vi "Parse Payload File.vi"(8 "error in":errorcluster, 11 "frame array path in":path caption="path to parameters xml") -> (0 "error out":errorcluster, 2 "Map":T1 {"value"."Type of Frame" items=["Raw Frame", "UDP/IP Tx Gen", "Tx UDP"]; "value"."Data" format="%.0x"}, 3 "frame array path out":path caption="path to parameters xml")   [LabVIEW 2020, in "AIM ARINC 664 Scripting.lvlib"]
uses:
  AIM ARINC 664 Scripting.lvlib
  Frame Configuration/controls/Type of Payload.ctl
  Frame Configuration/controls/Payload Record Type.ctl
  Frame Configuration/controls/Payload Map.ctl
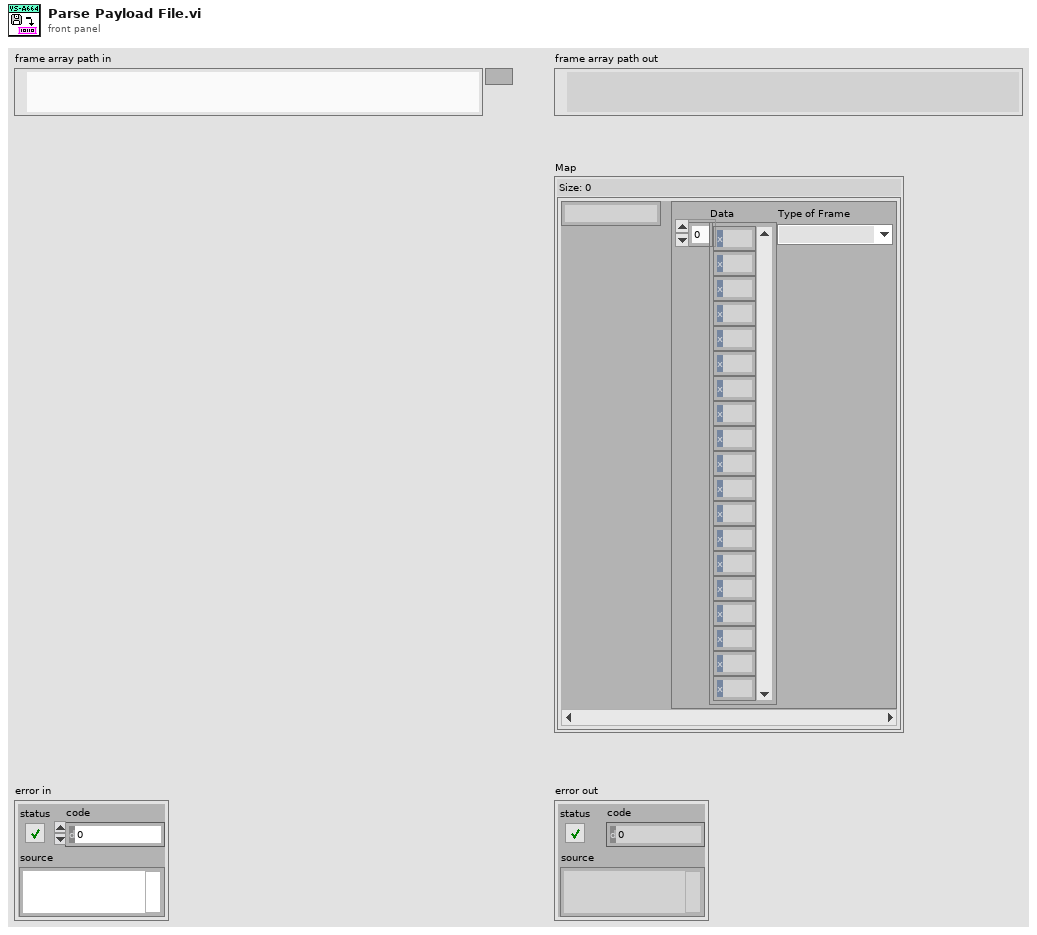
[diagram p1: front panel]
types:
  T1 = typedef "Payload Map.ctl" = map{string, T2}
  T2 = typedef "Payload Record Type.ctl" = cluster{"Data":u8[], "Type of Frame":T3}
  T3 = typedef "Type of Payload.ctl" = u16
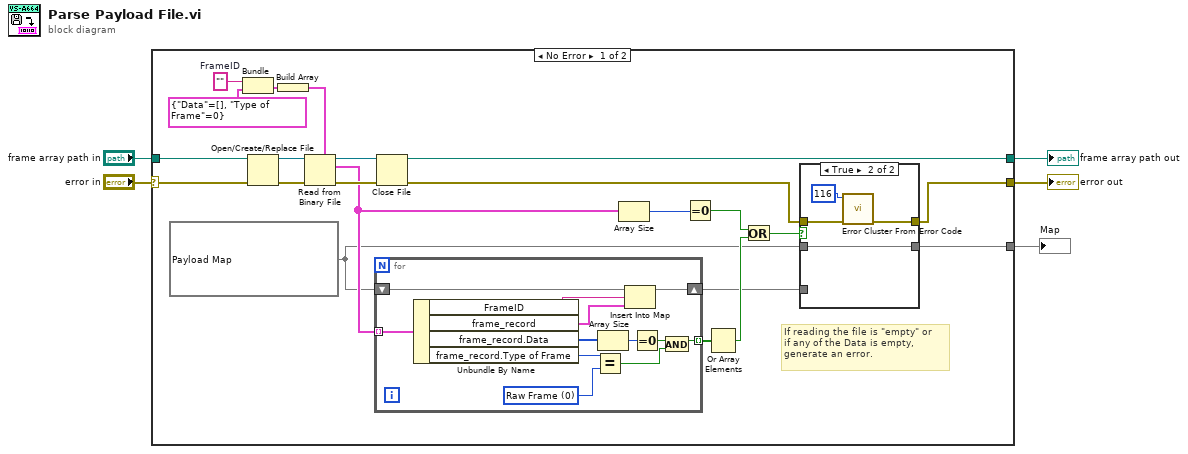
[diagram p0: block diagram]
diagram:
  n1 = case shown="No Error" "error in" {
    selector: "error in" -> [w22 w47]
    tunnel: [w15 w47] -> w5
    tunnel: "frame array path in" -> [w24 w46]
    tunnel: [w23 w46] -> w2
    tunnel: [w7 _] -> w1
    frame No Error {
      w20 = ""  # FrameID
      w6 = T1 {}
      # "If reading the file is \"empty\" or \nif any of the Data is empty,\ngenerate an error."
      n2 = Bundle("FrameID"=w20, "frame_record"=T2 {"Data"=[], "Type of Frame"=0}) -> (w21:cluster{"FrameID":string, "frame_record":T2})  [unwired: 1 in]
      n3 = Open/Create/Replace File(file path (use dialog)=w24, error in=w22) -> (refnum out=w26:refnum<file>, error out=w27:errorcluster)  [unwired: 4 in, 1 out]
      n4 = Build Array(w21) -> (w18:cluster{"FrameID":string, "frame_record":T2}[])
      n5 = Read from Binary File(5:w18, 8:w27, 11:w26) -> (0:w17:errorcluster, 2:w14:cluster{"FrameID":string, "frame_record":T2}[], 3:w25:refnum<file>)  [unwired: 3 in, 1 out]
      n6 = for {
        shift-right: [w44] -> w8
        shift-left: w6 -> [w45]
        tunnel: w14 -> [w41] mode=indexing
        tunnel: [w35] -> w10 mode=indexing
        w36 = T3 0 items=["Raw Frame", "UDP/IP Tx Gen", "Tx UDP"] ("y")
        n7 = Unbundle By Name(w41) -> ("FrameID"=w43:string, "frame_record"=w42:T2, "frame_record.Data"=w40:u8[], "frame_record.Type of Frame"=w37:T3)
        n8 = Equal?(x=w37, y=w36) -> (x = y?=w34:bool)
        n9 = Array Size(array=w40) -> (size(s)=w39:i32)
        n10 = Insert Into Map(map in=w45, key=w43, value=w42) -> (map out=w44:T1)  [unwired: 2 out]
        n11 = Equal To 0?(x=w39) -> (x = 0?=w38:bool)
        n12 = And(x=w38, y=w34) -> (x .and. y?=w35:bool)
      }
      n13 = Close File(refnum=w25, error in=w17) -> (path=w23:path, error out=w16:errorcluster)
      n14 = Array Size(array=w14) -> (size(s)=w13:i32)
      n15 = Equal To 0?(x=w13) -> (x = 0?=w12:bool)
      n16 = Or Array Elements(Boolean array=w10) -> (logical OR=w9:bool)
      n17 = Or(x=w12, y=w9) -> (x .or. y?=w11:bool)
      n18 = case shown="True" w11 {
        tunnel: w16 -> [w29 w33]
        tunnel: [w29 w32] -> w15
        tunnel: w8 -> [w28 _]
        tunnel: [w28 w30] -> w7
        tunnel: w6 -> [_ w30]
        frame False {
        }
        frame True {
          n19 = call <vilib>:"Error Cluster From Error Code.vi"("error in (no error)"=w33, "error code (0)"=116 ("t")) -> ("error out"=w32:errorcluster)  [unwired: 7 in]
        }
      }
    }
    frame Error {
    }
  }
  "error out" <- w5
  "frame array path out" <- w2
  "Map" <- w1
